vi "PH_SHS_Analysis_Calibrator.ProcPeriodic.vi"(0 "i ref in":refnum<vi>, 3 "ms timeout (100)":i32=100, 5 "error in (no error)":errorcluster) -> (14 "i ref out":refnum<vi>, 17 "timed out":bool, 19 "error out":errorcluster)   [LabVIEW 2014, in "PH_SHS_Analysis_Calibrator.lvlib"]
doc: "This method serves to periodically do things like reading values from the HW. Methods that should be executed periodically should be called from THIS methode. Add code here."
uses:
  PH_SHS_Analysis_Calibrator.lvlib
  PH_Img_BaseClass/PH_Img_BaseClass.lvlib
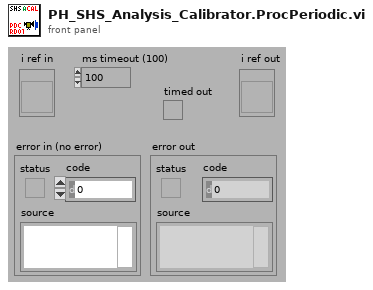
[diagram p1: front panel]
types:
  T1 = typedef "PH_Img_BaseClass.lvlib/PH_Img_BaseClass.i attribute.ctl" = cluster{"GUI Refs":T2, "Timeout Image [ms]":i32, "Default Periodic Period [ms]":i32, "Camera":cluster{"Instancename":string, "Notifier":refnum<notifier>}, "Palette":T3, "Cam Settings":cluster{"Cam ID":string, "Gain":dbl, "Brightness":dbl, "Shutter":dbl, "Cam Info Failure":bool, "Mode":i32}}
  T2 = typedef "PH_Img_BaseClass.lvlib/PH_Img_BaseClass.GUI Refs.ctl" = cluster{"Timeout":refnum<vi>, "Image":refnum<vi>, "Palette":refnum<vi>, "Timeout Set":refnum<vi>}
  T3 = typedef "PH_Img_BaseClass.lvlib/PH_Img_BaseClass.Palette.ctl" = i32
  T4 = typedef "IMAQ Image.ctl" = refnum<image>
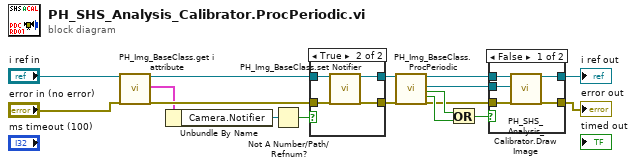
[diagram p0: block diagram]
diagram:
  n1 = call "PH_Img_BaseClass.get i attribute.vi"("i ref in"="i ref in", "error in (no error)"="error in (no error)") -> ("i ref out"=w14:refnum<vi>, "i attribute"=w15:T1, "error out"=w16:errorcluster)  [unwired: 15 in]
  n2 = Unbundle By Name(w15) -> ("Camera.Notifier"=w12:refnum<notifier>)
  n3 = Not A Number/Path/Refnum?(number/path/refnum=w12) -> (NaN/Path/Refnum?=w13:bool)
  n4 = case shown="True" w13 {
    tunnel: w16 -> [w19 w20]
    tunnel: w14 -> [w18 w23]
    tunnel: [w18 w22] -> w11
    tunnel: [w19 w21] -> w10
    frame False {
    }
    frame True {
      n5 = call "PH_Img_BaseClass.set Notifier.vi"("i ref in"=w23, "error in"=w20) -> ("i ref out"=w22:refnum<vi>, "error out"=w21:errorcluster)  [unwired: 16 in]
    }
  }
  n6 = call "PH_Img_BaseClass.ProcPeriodic.vi"("i ref in"=w11, "error in (no error)"=w10) -> ("i ref out"=w6:refnum<vi>, "Cam Image"=w1:T4, "timed out?"=w9:bool, "Error while unflatten data?"=w8:bool, "error out"=w7:errorcluster)  [unwired: 13 in]
  n7 = Or(x=w9, y=w8) -> (x .or. y?=w5:bool)
  n8 = case shown="False" w5 {
    tunnel: w6 -> [w28 w30]
    tunnel: [w25 w30] -> w17
    tunnel: w7 -> [w27 w29]
    tunnel: [w26 w29] -> w4
    tunnel: w1 -> [w24 _]
    frame False {
      n9 = call "PH_SHS_Analysis_Calibrator.Draw Image.vi"("i ref in"=w28, "Image"=w24, "error in (no error)"=w27) -> ("i ref out"=w25:refnum<vi>, "error out"=w26:errorcluster)  [unwired: 15 in]
    }
    frame True {
    }
  }
  "error out" <- w4
  "i ref out" <- w17
